vi "CalcFactor.vi"(6 "error in (no error)":errorcluster, 7 "delta":dbl, 8 "deltavec":dbl[](array[numeric]), 9 "point":dbl[](array[numeric])) -> (0 "error out":errorcluster, 3 "factor":dbl)   [LabVIEW 2010]
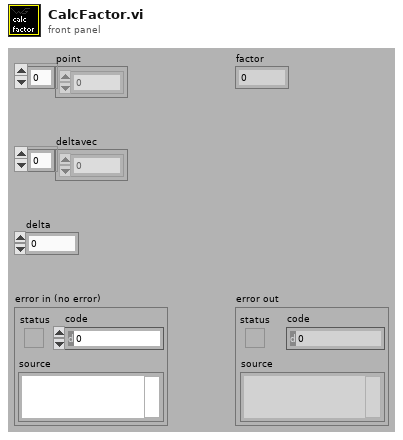
[diagram p1: front panel]
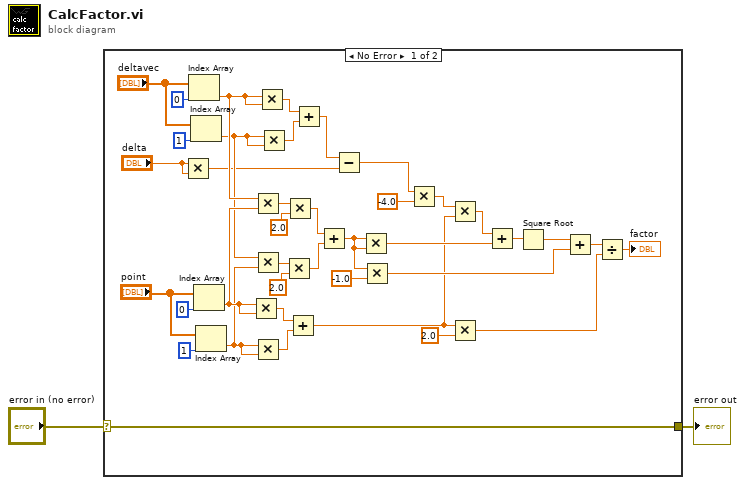
[diagram p0: block diagram]
diagram:
  n1 = case shown="No Error" "error in (no error)" {
    selector: "error in (no error)" -> [w3 w42]
    tunnel: [w3 w42] -> w1
    frame No Error {
      n2 = Multiply(x="delta", y="delta") -> (x*y=w4:dbl)
      n3 = Index Array(array="deltavec", index=0) -> (element=w30:dbl)
      n4 = Index Array(array="deltavec", index=1) -> (element=w27:dbl)
      n5 = Index Array(array="point", index=0) -> (element=w29:dbl)
      n6 = Index Array(array="point", index=1) -> (element=w28:dbl)
      n7 = Multiply(x=w29, y=w29) -> (x*y=w31:dbl)
      n8 = Multiply(x=w30, y=w29) -> (x*y=w23:dbl)
      n9 = Multiply(x=w27, y=w28) -> (x*y=w24:dbl)
      n10 = Multiply(x=w28, y=w28) -> (x*y=w32:dbl)
      n11 = Multiply(x=w30, y=w30) -> (x*y=w34:dbl)
      n12 = Multiply(x=w27, y=w27) -> (x*y=w35:dbl)
      n13 = Multiply(x=w24, y=2.0) -> (x*y=w21:dbl)
      n14 = Multiply(x=w23, y=2.0) -> (x*y=w22:dbl)
      n15 = Add(x=w31, y=w32) -> (x+y=w9:dbl)
      n16 = Add(x=w34, y=w35) -> (x+y=w33:dbl)
      n17 = Add(x=w22, y=w21) -> (x+y=w13:dbl)
      n18 = Subtract(x=w33, y=w4) -> (x-y=w19:dbl)
      n19 = Multiply(x=w13, y=w13) -> (x*y=w17:dbl)
      n20 = Multiply(x=w13, y=-1.0) -> (x*y=w12:dbl)
      n21 = Multiply(x=w19, y=-4.0) -> (x*y=w18:dbl)
      n22 = Multiply(x=w18, y=w9) -> (x*y=w16:dbl)
      n23 = Multiply(x=w9, y=2.0) -> (x*y=w8:dbl)
      n24 = Add(x=w16, y=w17) -> (x+y=w15:dbl)
      n25 = Square Root(x=w15) -> (sqrt(x)=w11:dbl)
      n26 = Add(x=w11, y=w12) -> (x+y=w7:dbl)
      n27 = Divide(x=w7, y=w8) -> (x/y=→"factor":dbl)
    }
    frame Error {
    }
  }
  "error out" <- w1
